vi "Read transmission data unit.vi"(8 "error in (no error)":errorcluster, 11 "Master CR in":refnum<class "Master CR.lvclass">) -> (0 "error out":errorcluster, 2 "Transmission Data Unit":refnum<class "Transmission Data Unit.lvclass">, 3 "Master CR out":refnum<class "Master CR.lvclass">)   [LabVIEW 2021]
uses:
  Master CR.lvclass
  Modbus_v121c/Network Protocol/Network Protocol.lvclass
  Modbus_v121c/Transmission Data Unit/Transmission Data Unit.lvclass
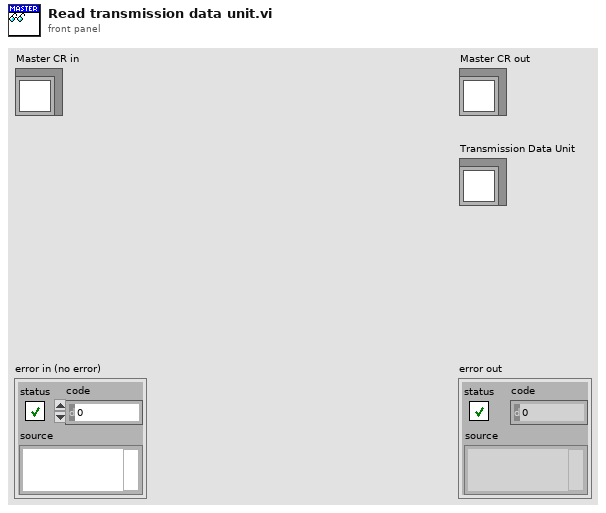
[diagram p1: front panel]
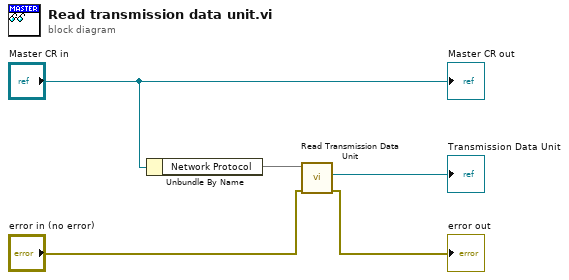
[diagram p0: block diagram]
diagram:
  n1 = Unbundle By Name("Master CR in") -> ("Network Protocol"=w4)
  n2 = call "Read Transmission Data Unit.vi"("error in (no error)"="error in (no error)", "Network Protocol in"=w4) -> ("error out"=→"error out":errorcluster, "Transmission Data Unit"=→"Transmission Data Unit":refnum<class "Transmission Data Unit.lvclass">)  [unwired: 7 in, 1 out]
  "Master CR out" <- "Master CR in"
